vi "PopulateProbe.vi"(8 "error in (no error)":errorcluster, 10 "Multicolumn Listbox in":refnum<vi>, 11 "LinkedList in":refnum<class "LinkedList.lvclass">) -> (0 "error out":errorcluster, 2 "Multicolumn Listbox out":refnum<vi>, 3 "LinkedList out":refnum<class "LinkedList.lvclass">)   [LabVIEW 2009, in "LinkedList.lvclass"]
uses:
  LinkedList.lvclass
  LLNode/LLNode.lvclass
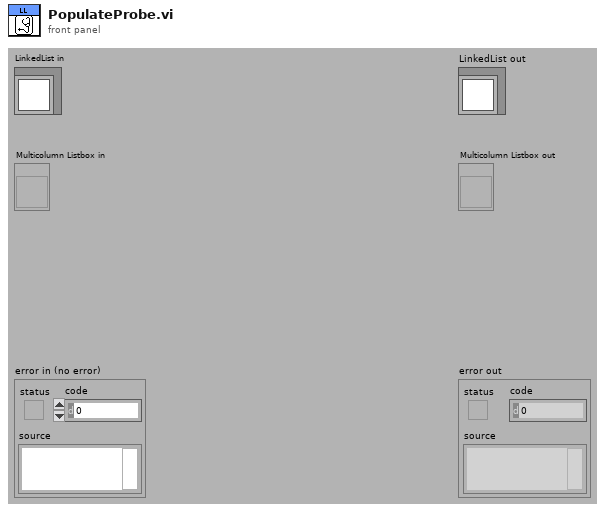
[diagram p1: front panel]
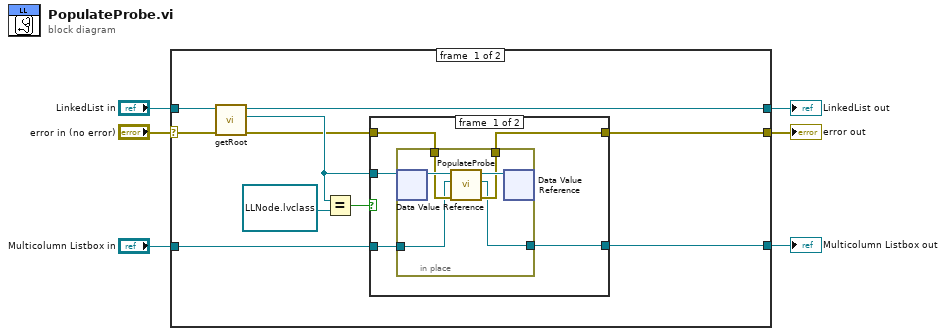
[diagram p0: block diagram]
diagram:
  n1 = case shown="No Error" "error in (no error)" {
    selector: "error in (no error)" -> [w14 w32]
    tunnel: [w9 w32] -> w5
    tunnel: [w15 w31] -> w3
    tunnel: "LinkedList in" -> [w16 w31]
    tunnel: "Multicolumn Listbox in" -> [w8 w30]
    tunnel: [w7 w30] -> w1
    frame #0 {
      n2 = call "getRoot.vi"("error in (no error)"=w14, "LinkedList in"=w16) -> ("error out"=w10:errorcluster, "Root"=w11:refnum<data-value>, "LinkedList out"=w15:refnum<class "LinkedList.lvclass">)  [unwired: 7 in]
      n3 = Equal?(x=w11, y=refnum<data-value> refnum) -> (x = y?=w12:bool)
      n4 = case shown="False" w12 {
        tunnel: w11 -> [w21 _]
        tunnel: w10 -> [w20 w29]
        tunnel: [w19 w29] -> w9
        tunnel: w8 -> [w18 w28]
        tunnel: [w17 w28] -> w7
        frame #0 {
          n5 = in-place {
            in-place-border: w20 -> [w25]
            in-place-border: [w24] -> w19
            in-place-border: w18 -> [w23]
            in-place-border: [w22] -> w17
            n6 = in-place-dvr #1(w21) -> (w27:refnum<class "LLNode.lvclass">)  [unwired: 1 out]
            n7 = call-dynamic "PopulateProbe.vi"("error in (no error)"=w25, "Multicolumn Listbox in"=w23, "LLNode in"=w27) -> ("error out"=w24:errorcluster, "Multicolumn Listbox out"=w22:refnum<vi>, "LLNode out"=w26:refnum<class "LLNode.lvclass">)  [unwired: 6 in]
            n8 = in-place-dvr #1(w26) -> ()  [unwired: 2 out]
          }
        }
        frame #1 {
        }
      }
    }
    frame #1 {
    }
  }
  "error out" <- w5
  "LinkedList out" <- w3
  "Multicolumn Listbox out" <- w1
